vi "Init.vi"(6 "Post Meas?":bool, 7 "Prepend Result Name":bool, 8 "error in (no error)":errorcluster, 9 "Measurement Name":string, 10 "SA Pin":string, 11 "Standard":string) -> (0 "error out":errorcluster, 3 "PAE out":refnum<class "PAE.lvclass">)   [LabVIEW 2016, in "SeqAuto Evaluations.lvlib" / "PAE.lvclass"]
uses:
  PAE.lvclass
  C:/Sequence Automation/Plugins/SeqAuto IEvaluation.lvlibp/SeqAuto IEvaluation.lvclass
  PAE.lvclass/PAE.ctl
  Write SA Pin.vi
  Plugins/SeqAuto IEvaluation.lvlibp/Write Measurement Name.vi
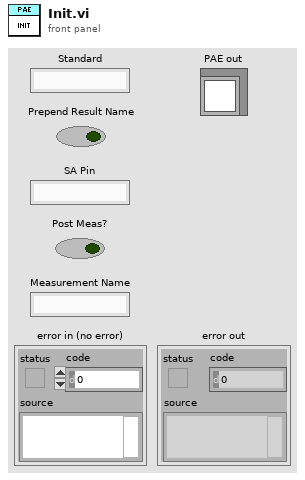
[diagram p1: front panel]
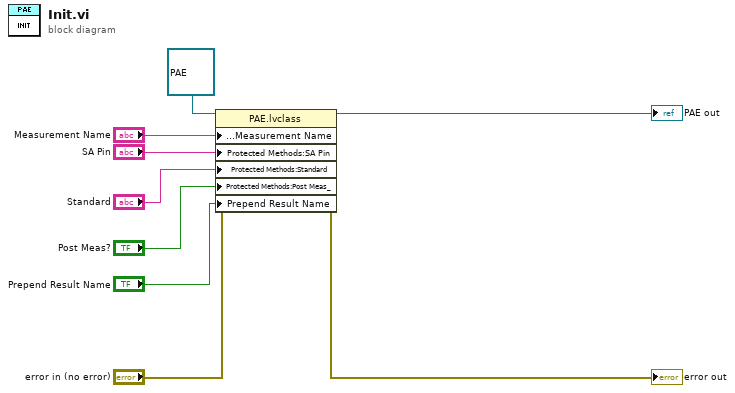
[diagram p0: block diagram]
diagram:
  n1 = property class="PAE.lvclass"(reference=refnum<class "PAE.lvclass"> refnum ("PAE in"), error in="error in (no error)", "Protected Methods:Measurement Name"="Measurement Name", "Protected Methods:SA Pin"="SA Pin", "Protected Methods:Standard"="Standard", "Protected Methods:Post Meas_"="Post Meas?", "Prepend Result Name"="Prepend Result Name") -> (reference out=→"PAE out":refnum<class "PAE.lvclass">, error out=→"error out":errorcluster)
